vi "Muxed_Stream_1channel.vi"() -> ()   [LabVIEW 2014]
uses:
  <vilib>/FPGAPlugInAG/PXI-7852R/niLvFpga_Open_PXI-7852R.vi
  <vilib>/rvi/interface/common/dynamic/niFpgaDynamicAddResources.vi
  <vilib>/Utility/error.llb/Error Cluster From Error Code.vi
  <vilib>/rvi/errors/niLvFpgaAdjustHostInterfaceError.vi
  <vilib>/measure/maspectr.llb/FFT Power Spectrum and PSD for 1 Chan.vi
  <vilib>/Utility/file.llb/Write To Spreadsheet File (I64).vi
  <vilib>/FPGAPlugInAG/Dynamic/niLvFpga_Close_Dynamic.vi
  <vilib>/rvi/interface/nirviOpenFPGA/nirviOpenFPGA.xnode
  FPGA Bitfiles/MilitaruDAQ_FPGATarget_MuxedAcquisition_p8S6tR+nlj8.lvbitx
  Muxed_Acquisition_1channel.vi
  <vilib>/rvi/interface/nirviReadWriteControl/nirviReadWriteControl.xnode
  <vilib>/rvi/interface/nirviMethod/nirviMethod.xnode
  <vilib>/rvi/interface/nirviCloseFPGA/nirviCloseFPGA.xnode
  <vilib>/measure/NI_MAPro.lvlib
  <vilib>/rvi/interface/Simulation/niFpgaSimulationCallBeginRW.vi
  NiFpgaLv.dll
  <vilib>/FPGAPlugInAG/Dynamic/niLvFpga_ReadFifo_Dynamic.vi
  <vilib>/rvi/errors/niLvFpgaMergeErrorWithErrorCode.vi
panel:
  in  "Acquisition-Channel":i16
  out "FIFO timeout":bool
  out "Acquisition Timeout":bool
  out "Sampling Frequency\n(kHz)":dbl
  in  "Sampling(Ticks)":u32
  in  "Number of Elements":u32
  out "Position":waveform(i16)(graph) caption="Dynamic Data Type"
  in  "dB On (F)":bool
  in  "averaging parameters":T1={"averaging mode"=enum."No averaging", "weighting mode"=enum."Exponential", "number of averages"=10} {"number of averages" min=1}
  out "PSD":cluster{"f0":dbl, "df":dbl, "magnitude":dbl[]}(graph) caption="Dynamic Data Type"
  in  "file path (dialog if empty)":path
  in  "append to file? (new file:F)":bool
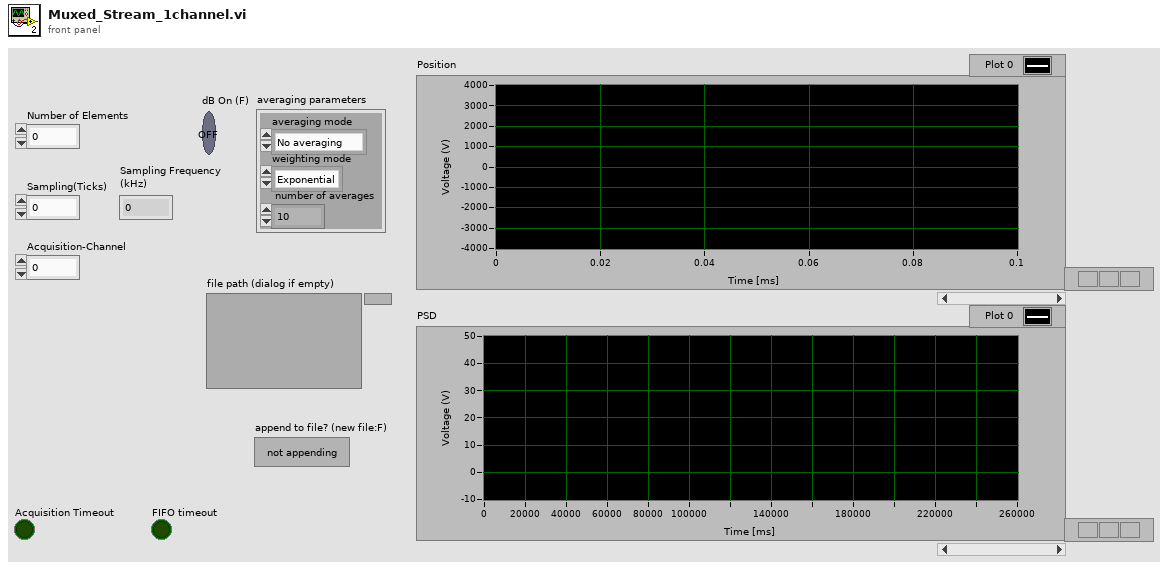
[diagram p1: front panel]
types:
  T1 = cluster{"averaging mode":enum16{"No averaging", "Vector averaging", "RMS averaging", "Peak hold"}, "weighting mode":enum16{"Linear", "Exponential"}, "number of averages":u32}
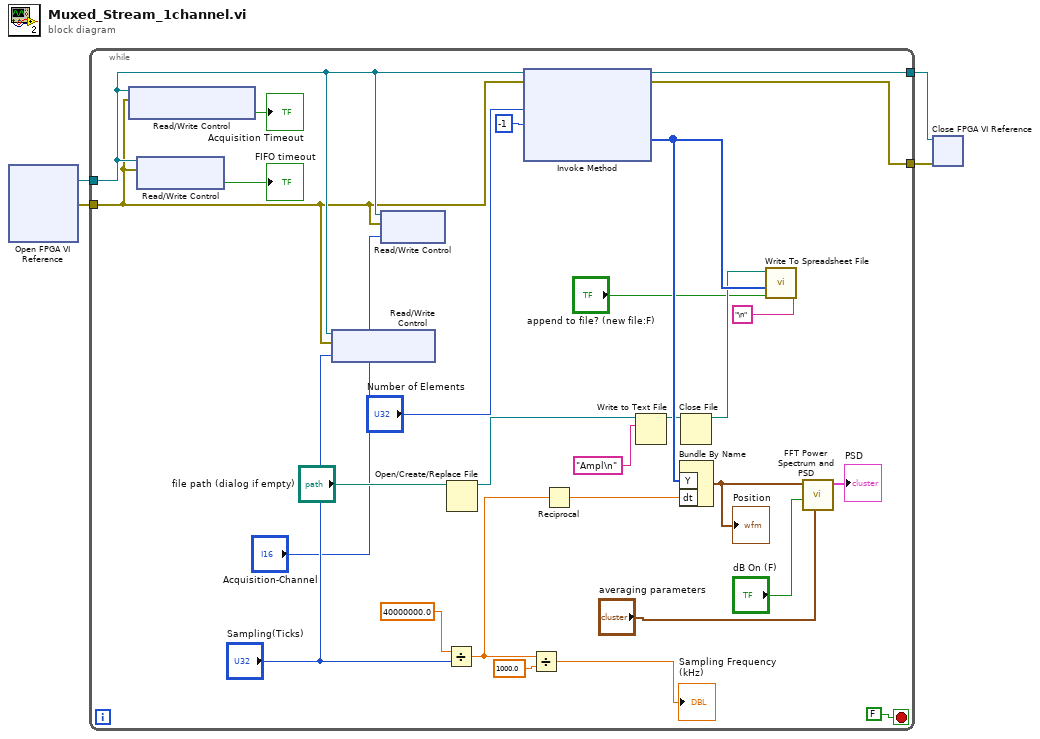
[diagram p0: block diagram]
diagram:
  n1 = xnode "Open FPGA VI Reference"() -> ("FPGA VI Reference Out"=w4:refnum<k20>, "error out"=w3:errorcluster)  [unwired: 2 in]
  n2 = while {
    tunnel: w4 -> [w10]
    tunnel: w3 -> [w9]
    tunnel: [w25] -> w1
    tunnel: [w24] -> w2
    stop <- FALSE stop-if-true
    n3 = xnode "Read/Write Control"("FPGA VI Reference In"=w10, "error in"=w9) -> ("Acquisition Timeout"=→"Acquisition Timeout":bool)  [unwired: 2 out]
    n4 = xnode "Read/Write Control"("FPGA VI Reference In"=w10, "error in"=w9) -> ("FIFO timeout"=→"FIFO timeout":bool)  [unwired: 2 out]
    n5 = xnode "Read/Write Control"("FPGA VI Reference In"=w10, "error in"=w9, "Sampling(Ticks)"="Sampling(Ticks)") -> ()  [unwired: 2 out]
    n6 = xnode "Read/Write Control"("FPGA VI Reference In"=w10, "error in"=w9, "Numeric"="Acquisition-Channel") -> ()  [unwired: 2 out]
    n7 = Divide(x=40000000.0, y="Sampling(Ticks)") -> (x/y=w6:dbl)
    n8 = Open/Create/Replace File(file path (use dialog)="file path (dialog if empty)") -> (refnum out=w19:refnum<file>)  [unwired: 5 in, 2 out]
    n9 = xnode "Invoke Method"("FPGA VI Reference In"=w10, "error in"=w9, "Number of Elements"="Number of Elements", "Timeout (ms)"=-1) -> ("FPGA VI Reference Out"=w25:refnum<k20>, "error out"=w24:errorcluster, "Data"=w23:i16[])  [unwired: 1 out]
    n10 = Divide(x=w6, y=1000.0) -> (x/y=→"Sampling Frequency\n(kHz)":dbl)
    n11 = Reciprocal(x=w6) -> (1/x=w13:dbl)
    n12 = Write to Text File(file (use dialog)=w19, text="Ampl\n") -> (refnum out=w18:refnum<file>)  [unwired: 2 in, 2 out]
    n13 = Bundle By Name ("Build Waveform")("Y"=w23, "dt"=w13) -> (w29:waveform(i16))  [unwired: 1 in]
    "Position" <- w29
    n14 = Close File(refnum=w18) -> (path=w17:path)  [unwired: 1 in, 1 out]
    n15 = call-poly <vilib>:"Write To Spreadsheet File.vi"("delimiter (\\t)"="\n" ("delimiter (\\t)"), "append to file? (new file:F)"="append to file? (new file:F)", "1D data"=w23, "file path (dialog if empty)"=w17) -> ()  [unwired: 4 in, 1 out]
    n16 = call-poly <vilib>:"FFT Power Spectrum and PSD.vi"("averaging parameters"="averaging parameters", "dB On (F)"="dB On (F)", "time signal"=w29) -> ("Power Spectrum / PSD"=→"PSD":cluster{"f0":dbl, "df":dbl, "magnitude":dbl[]})  [unwired: 5 in, 3 out]
  }
  n17 = xnode "Close FPGA VI Reference"("FPGA VI Reference In"=w1, "error in"=w2) -> ()  [unwired: 1 out]
